vi "case_request_data.vi"(5 "Uninitialized message":string, 7 "initialized":bool, 8 "error in (no error)":errorcluster, 10 "This VI":refnum<vi>, 11 "VISA resource name in":refnum<visa-resource-name>) -> (0 "error out":errorcluster, 3 "VISA Refnum out":refnum<visa-resource-name>)   [LabVIEW 2020]
uses:
  c517460c-609a-47ee-bb93-6f9d2f0c314d.vi
  12185cb5-c390-449e-a567-8e93b21409db.vi
  e36c5e91-f142-4194-84c7-f86b29cd7bc4.vi
  <instrlib>/Marlin Instrument Driver/Marlin Instrument Driver.lvlib
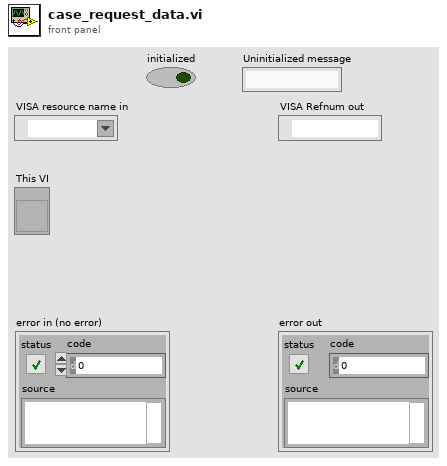
[diagram p1: front panel]
types:
  T1 = typedef "Marlin Instrument Driver.lvlib/end stop status.ctl" = cluster{"x_min":bool, "y_min":bool, "z_min":bool}
  T2 = typedef "Marlin Instrument Driver.lvlib/temperatures.ctl" = cluster{"T":dbl, "T setpoint":dbl, "B":dbl, "B setpoint":dbl}
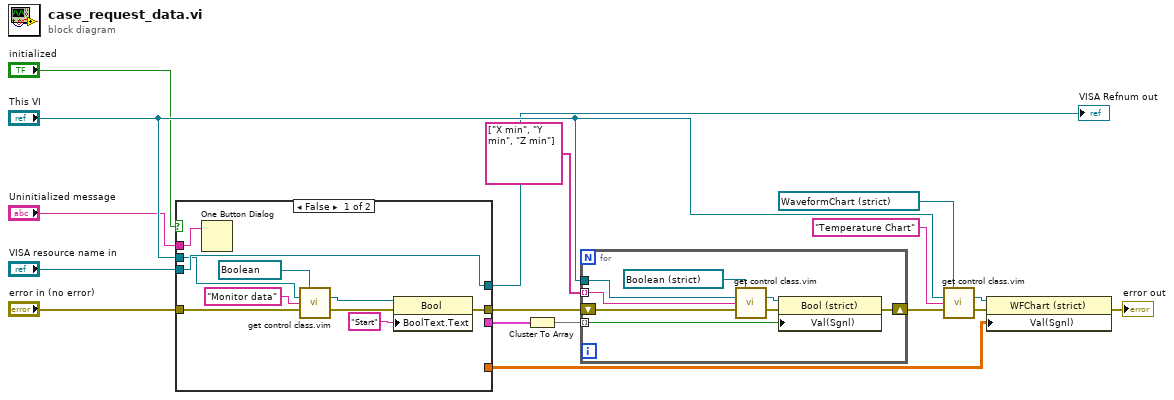
[diagram p0: block diagram]
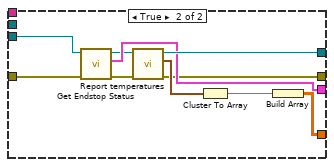
[diagram p2: hidden frame]
diagram:
  n1 = case shown="False" "initialized" {
    tunnel: "VISA resource name in" -> [w27 w37]
    tunnel: [w27 w36] -> w2
    tunnel: [_ w35] -> w7
    tunnel: [_ w30] -> w15
    tunnel: "error in (no error)" -> [w20 w29]
    tunnel: [w19 w28] -> w9
    tunnel: "Uninitialized message" -> [w26 _]
    tunnel: "This VI" -> [w18 _]
    frame False {
      n2 = One Button Dialog(message=w26) -> ()  [unwired: 1 in, 1 out]
      n3 = call "get control class.vim"("Control class"=refnum<vi> refnum ("reference out"), "Main VI reference"=w18, "Label"="Monitor data", "error in (no error)"=w20) -> ("Control out"=w22:refnum<vi>, "error out"=w21:errorcluster)  [unwired: 10 in]
      n4 = property on="Property Node" class="Bool"(reference=w22, error in=w21, "BoolText.Text"="Start" ("Boolean Text.Text")) -> (error out=w19:errorcluster)  [unwired: 1 out]
    }
    frame True {
      n5 = call <instrlib>:"Get Endstop Status.vi"("error in (no error)"=w29, "VISA resource name"=w37) -> ("error out"=w32:errorcluster, "End stop status"=w35:T1, "VISA resource name out"=w34:refnum<visa-resource-name>)  [unwired: 7 in]
      n6 = call <instrlib>:"Report temperatures.vi"("error in (no error)"=w32, "VISA resource name"=w34) -> ("error out"=w28:errorcluster, "Temperatures"=w33:T2, "VISA resource name out"=w36:refnum<visa-resource-name>)  [unwired: 7 in]
      n7 = Cluster To Array(cluster=w33) -> (array=w31:dbl[])
      n8 = Build Array(w31) -> (w30:dbl[][])
    }
  }
  "VISA Refnum out" <- w2
  n9 = Cluster To Array(cluster=w7) -> (array=w8:bool[])
  n10 = for {
    tunnel: string[] ["X min", "Y min", "Z min"] -> [w45] mode=indexing
    tunnel: w8 -> [w43] mode=indexing
    shift-right: [w39] -> w16
    shift-left: w9 -> [w40]
    tunnel: "This VI" -> [w38]
    n11 = call "get control class.vim"("Control class"=refnum<vi> refnum ("Z min"), "Main VI reference"=w38, "Label"=w45, "error in (no error)"=w40) -> ("Control out"=w42:refnum<vi>, "error out"=w41:errorcluster)  [unwired: 10 in]
    n12 = property on="Property Node" class="Bool (strict)"(reference=w42, error in=w41, "Val(Sgnl)"=w43) -> (error out=w39:errorcluster)  [unwired: 1 out]
  }
  n13 = call "get control class.vim"("Control class"=refnum<vi> refnum ("Temperature Chart"), "Main VI reference"="This VI", "Label"="Temperature Chart", "error in (no error)"=w16) -> ("Control out"=w13:refnum<vi>, "error out"=w14:errorcluster)  [unwired: 10 in]
  n14 = property on="Property Node" class="WFChart (strict)"(reference=w13, error in=w14, "Val(Sgnl)"=w15) -> (error out=→"error out":errorcluster)  [unwired: 1 out]
